vi "Transfer image from FPGA to RT (SubVI).vi"(6 "Timeout (ms)":i32=5000, 9 "Image Size in":T2={"Rows (X)"=256, "Colums (Y)"=256}, 10 "Image In":T3, 11 "Refnum in":T1) -> (1 "Image Size out":T2={"Rows (X)"=256, "Colums (Y)"=256}, 2 "Image out":T3, 3 "Refnum out":T1)   [LabVIEW 2025, in "SoC IP Library.lvlib"]
uses:
  SoC IP Library.lvlib
  <vilib>/vision/Image Controls.llb/IMAQ Image.ctl
  Controls/Image Size.ctl
  Controls/FPGA Reference Type.ctl
  <vilib>/Utility/error.llb/Error Cluster From Error Code.vi
  <vilib>/rvi/errors/niLvFpgaAdjustHostInterfaceError.vi
  <vilib>/rvi/interface/nirviMethod/nirviMethod.xnode
  <vilib>/FPGAPlugInAG/Dynamic/niLvFpga_ReadFifo_Dynamic.vi
  <vilib>/rvi/errors/niLvFpgaMergeErrorWithErrorCode.vi
  <vilib>/vision/NI_Vision_Development_Module.lvlib
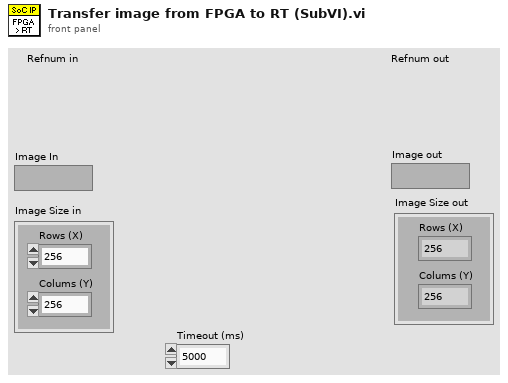
[diagram p1: front panel]
types:
  T1 = typedef "SoC IP Library.lvlib/FPGA Reference Type.ctl" = refnum<k20>
  T2 = typedef "SoC IP Library.lvlib/Image Size.ctl" = cluster{"Rows (X)":u16, "Colums (Y)":u16}
  T3 = typedef "IMAQ Image.ctl" = refnum<image>
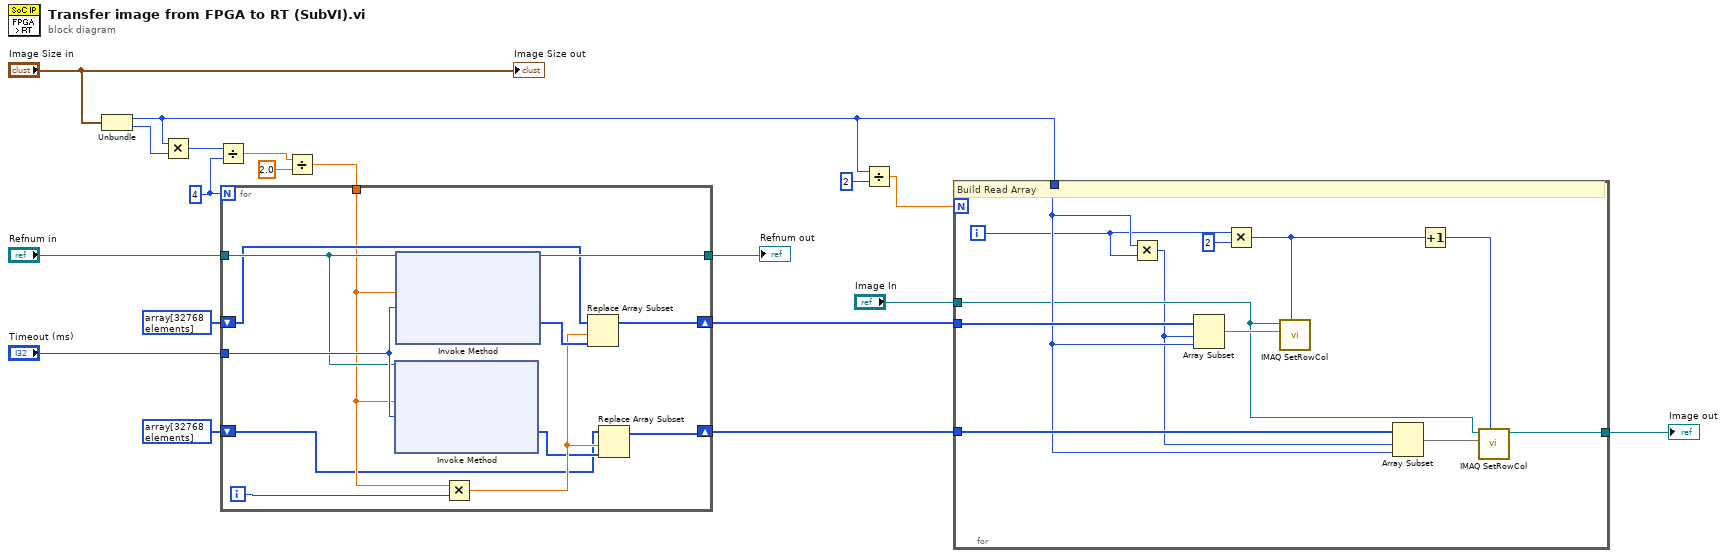
[diagram p0: block diagram]
diagram:
  w13 = 4
  n1 = Unbundle("Image Size in") -> ("Rows (X)"=w6:u16, "Colums (Y)"=w5:u16)
  n2 = Multiply(x=w6, y=w5) -> (x*y=w12:u32)
  n3 = Divide(x=w12, y=w13) -> (x/y=w8:dbl)
  n4 = Divide(x=w8, y=2.0) -> (x/y=w14:dbl)
  n5 = for {
    N: w13 -> [_]
    tunnel: w14 -> [w25]
    tunnel: "Refnum in" -> [w30]
    tunnel: "Timeout (ms)" -> [w31]
    tunnel: [w29] -> w1
    shift-right: [w27] -> w11
    shift-left: u8[] array[32768 elements] ("Data") -> [w28]
    shift-right: [w20] -> w10
    shift-left: u8[] array[32768 elements] ("Data") -> [w21]
    i -> [w24]
    n6 = xnode "Invoke Method"("FPGA VI Reference In"=w30, "Number of Elements"=w25, "Timeout (ms)"=w31) -> ("Data"=w22:u8[])  [unwired: 1 in, 3 out]
    n7 = xnode "Invoke Method"("FPGA VI Reference In"=w30, "Number of Elements"=w25, "Timeout (ms)"=w31) -> ("FPGA VI Reference Out"=w29:T1, "Data"=w26:u8[])  [unwired: 1 in, 2 out]
    n8 = Multiply(x=w25, y=w24) -> (x*y=w23:dbl)
    n9 = Replace Array Subset(array=w28, new element=w26, index=w23) -> (w27:u8[])
    n10 = Replace Array Subset(array=w21, new element=w22, index=w23) -> (w20:u8[])
  }
  "Refnum out" <- w1
  n11 = Divide(x=w6, y=u16 2) -> (x/y=w17:dbl)
  n12 = for {
    N: w17 -> [_]
    tunnel: w10 -> [w43]
    tunnel: w11 -> [w42]
    tunnel: "Image In" -> [w38]
    tunnel: w6 -> [w39]
    tunnel: [w32] -> w19
    i -> [w37]
    # "Build Read Array"
    n13 = Multiply(x=w39, y=w37) -> (x*y=w36:i32)
    n14 = Array Subset(array=w42, index=w36, length=w39) -> (w41:u8[])
    n15 = Multiply(x=w37, y=2) -> (x*y=w34:i32)
    n16 = call "IMAQ SetRowCol"("Number"=w34, "Pixels (U8)"=w41, "Image"=w38) -> ()  [unwired: 7 in, 2 out]
    n17 = Array Subset(array=w43, index=w36, length=w39) -> (w40:u8[])
    n18 = Increment(x=w34) -> (x+1=w33:i32)
    n19 = call "IMAQ SetRowCol"("Number"=w33, "Pixels (U8)"=w40, "Image"=w38) -> ("Image Out"=w32:T3)  [unwired: 7 in, 1 out]
  }
  "Image out" <- w19
  "Image Size out" <- "Image Size in"
